vi "Create Command.vi"(8 "error in (no error)":errorcluster, 11 "Message Channel in":T1 format="%.0x") -> (0 "error out":errorcluster, 3 "Message Channel out":T1 format="%.0x")   [LabVIEW 2018, in "Instrument Addon Scripting API.lvlib"]
uses:
  Instrument Addon Scripting API.lvlib
  <vilib>/NI Veristand/Custom Device API/Custom Device Item Ref.ctl
  Addon/Addon Shared/SubVIs/Constants.vi
  Addon/Addon Shared/Instrument Addon Shared.lvlib
  <vilib>/NI Veristand/Custom Device API/Custom Device API.lvlib
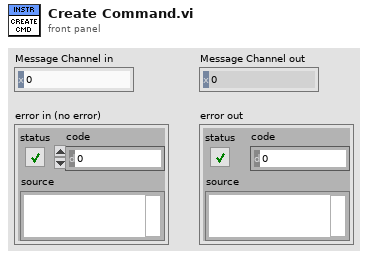
[diagram p1: front panel]
types:
  T1 = typedef "Custom Device API.lvlib/Custom Device Item Ref.ctl" = u64
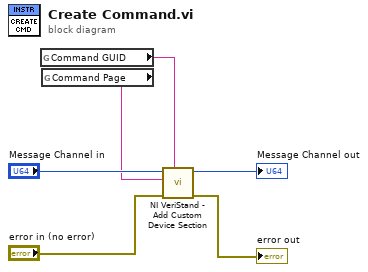
[diagram p0: block diagram]
diagram:
  n1 = global read "Constants.vi" "Command GUID"() -> (w1:string)
  n2 = global read "Constants.vi" "Command Page"() -> (w2:string)
  n3 = call <vilib>:"NI VeriStand - Add Custom Device Section.vi"("GUID (Default Section)"=w1, "error in (no error)"="error in (no error)", "Section Name"=w2, "Parent Ref in"="Message Channel in") -> ("error out"=→"error out":errorcluster, "Parent Ref out"=→"Message Channel out":T1)  [unwired: 4 in, 2 out]
